vi "z reply replier id.vi"(8 "error in (no error)":errorcluster, 10 "out_id":cluster{}, 11 "this_":cluster{}) -> (0 "error out":errorcluster, 2 "out_id out":cluster{}, 3 "function return":bool)   [LabVIEW 2021, in "zenohc.lvlib"]
doc: "bool z_reply_replier_id(const struct z_loaned_reply_t *this_,\n struct z_entity_global_id_t *out_id);"
uses:
  zenohc.lvlib
  zenohc.dll
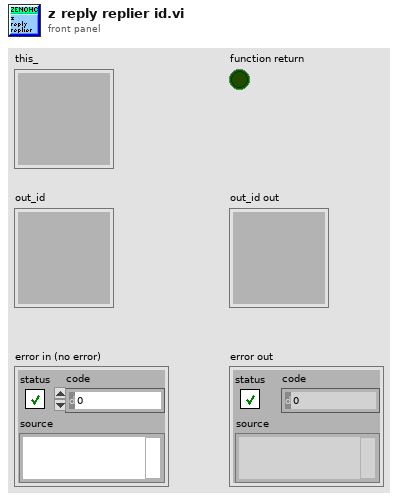
[diagram p1: front panel]
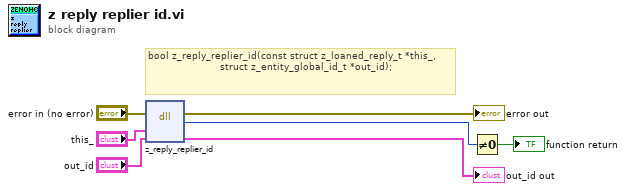
[diagram p0: block diagram]
diagram:
  # "bool z_reply_replier_id(const struct z_loaned_reply_t *this_,\n                        struct z_entity_global_id_t *out_id);"
  n1 = dll-call lib="D:/dev/zenoh_labview/zenohc/zenohc.*" fn="z_reply_replier_id"(error in="error in (no error)", "this_"="this_", "out_id"="out_id") -> (error out=→"error out":errorcluster, w6:u8, "out_id"=→"out_id out":cluster{})  [unwired: 3 in, 1 out]
  n2 = Not Equal To 0?(x=w6) -> (x != 0?=→"function return":bool)
